vi "EON SubVI.vi"(0 "Image":T1, 5 "Coord details":T2, 7 "Calibrated Image":T1, 11 "error in (no error)":errorcluster, 12 "M ROI":T3) -> (4 "Image Out":T1, 6 "EON outer width":sgl format="%.2f", 8 "EON Presence/Absence":bool, 15 "error out":errorcluster)   [LabVIEW 2019, in "Algorithm.lvclass"]
uses:
  FrameworkOverrides/Algorithm.lvclass
  <vilib>/vision/NI_Vision_Development_Module.lvlib
  <vilib>/vision/Measure.llb/Edge Polarity.ctl
  <vilib>/vision/Measure.llb/Edge Options.ctl
  <vilib>/vision/Image Controls.llb/IMAQ Image.ctl
panel:
  out "Overlay Delay":u64
  out "EON Presence":i32
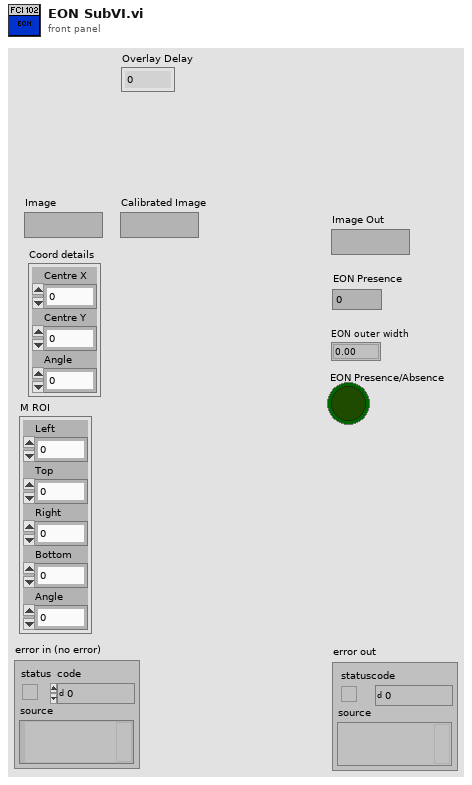
[diagram p1: front panel]
types:
  T1 = typedef "IMAQ Image.ctl" = refnum<image>
  T2 = cluster{"Centre X":dbl, "Centre Y":dbl, "Angle":dbl}
  T3 = cluster{"Left":dbl, "Top":dbl, "Right":dbl, "Bottom":dbl, "Angle":dbl}
  T4 = typedef "Edge Options.ctl" = cluster{"Edge Polarity":T5, "Kernel Size":u32, "Width":u32, "Minimum Edge Strength":sgl, "Interpolation Type":enum32{"Zero Order", "Bilinear", "Quadratic", "Cubic", "Bilinear Fixed"}, "Data Processing Method":enum32{"Average", "Median"}}
  T5 = typedef "Edge Polarity.ctl" = u32
  T6 = typedef "Particle Parameters" = i32
  T7 = cluster{"Measurement Parameter":T6, "Range Lower Value":dbl, "Range Upper Value":dbl, "Range":bool, "Measurement Type":bool}[]
  T8 = typedef "Image Type" = u32
  T9 = typedef "ROI Descriptor" = cluster{"Global Rectangle":i32[], "Contours":cluster{"ID":enum32{"External", "Internal"}, "Type":u32, "Coordinates":i32[]}[]}
  T10 = typedef "Search Line.ctl" = cluster{"Start Point":cluster{"X":sgl, "Y":sgl}, "End Point":cluster{"X":sgl, "Y":sgl}, "Edge Info":T11[], "Edge Map":dbl[], "Calibration Valid":bool}
  T11 = typedef "Edge New.ctl" = cluster{"Location (Pixel)":cluster{"X":sgl, "Y":sgl}, "Location (Real-World)":cluster{"X":sgl, "Y":sgl}, "Distance (Pixel)":dbl, "Distance (Real-World)":dbl, "Strength":dbl, "Noise":dbl, "Rising?":bool}
  T12 = cluster{"Search Lines":T10[], "First Edge Points Array":cluster{"X":sgl, "Y":sgl}[], "Last Edge Points Array":cluster{"X":sgl, "Y":sgl}[]}
  T13 = cluster{"First Edge Point":cluster{"X":sgl, "Y":sgl}, "Search Line First Edge":cluster{"X":sgl, "Y":sgl}}
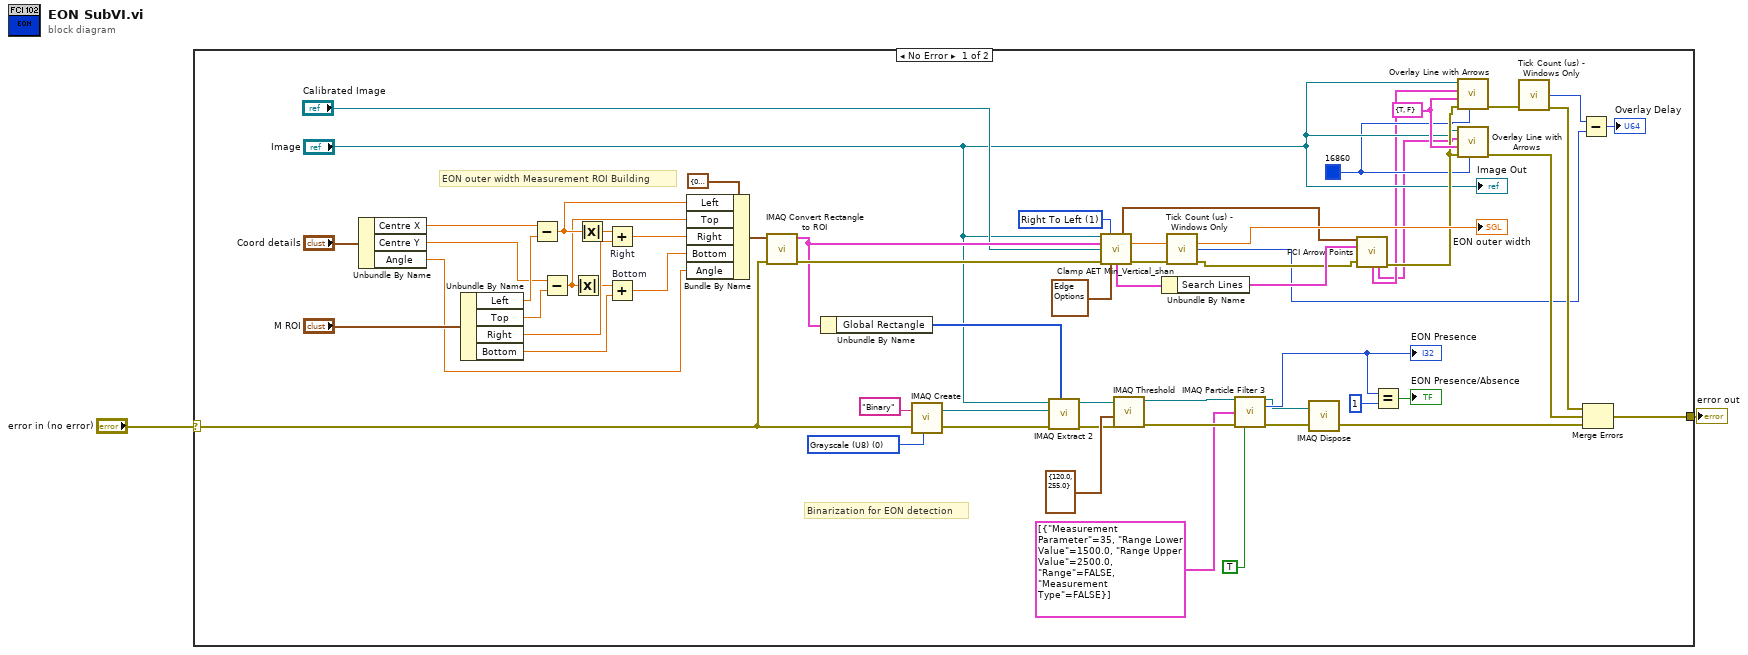
[diagram p0: block diagram]
diagram:
  n1 = case shown="No Error" "error in (no error)" {
    selector: "error in (no error)" -> [w22 w63]
    tunnel: [w21 w63] -> w1
    frame No Error {
      w13 = u32 16860 ("Color")
      w18 = cluster{"Start point":bool, "End point":bool} {"Start point"=TRUE, "End point"=FALSE} ("Arrows")
      w37 = T8 0 items=["Grayscale (U8)", "Grayscale (I16)", "Grayscale (SGL)", "Complex (CSG)", "RGB (U32)", "HSL (U32)", "RGB (U64)", "Grayscale (U16)"] ("Image Type")
      w49 = u16 1 items=["Left To Right", "Right To Left", "Top To Bottom", "Bottom To Top"] ("Scanning axis")
      # "Binarization for EON detection"
      # "EON outer width Measurement ROI Building"
      n2 = Unbundle By Name("Coord details") -> ("Centre X"=w25:dbl, "Centre Y"=w24:dbl, "Angle"=w23:dbl)
      n3 = Unbundle By Name("M ROI") -> ("Left"=w57:dbl, "Top"=w56:dbl, "Right"=w55:dbl, "Bottom"=w54:dbl)
      n4 = Subtract(x=w25, y=w57) -> (x-y=w60:dbl)
      n5 = Subtract(x=w24, y=w56) -> (x-y=w52:dbl)
      n6 = Absolute Value(x=w52) -> (abs(x)=w53:dbl)
      n7 = Absolute Value(x=w60) -> (abs(x)=w62:dbl)
      n8 = Add "Right"(x=w62, y=w55) -> (x+y=w59:dbl)
      n9 = Add "Bottom"(x=w53, y=w54) -> (x+y=w58:dbl)
      n10 = Bundle By Name(cluster=T3 {"Left"=0.0, "Top"=0.0, "Right"=0.0, "Bottom"=0.0, "Angle"=0.0} ("input cluster"), "Left"=w60, "Top"=w52, "Right"=w59, "Bottom"=w58, "Angle"=w23) -> (w51:T3)
      n11 = call "IMAQ Convert Rectangle to ROI"("error in (no error)"=w22, "Rectangle"=w51) -> ("error out"=w50:errorcluster, "ROI Descriptor"=w43:T9)  [unwired: 7 in]
      n12 = Unbundle By Name(w43) -> ("Global Rectangle"=w42:i32[])
      n13 = call "IMAQ Create"("Image Name"="Binary", "Image Type"=w37, "error in (no error)"=w22) -> ("New Image"=w28:T1, "error out"=w33:errorcluster)  [unwired: 2 in]
      n14 = call "IMAQ Extract 2"("Optional Rectangle"=w42, "error in (no error)"=w33, "Image Dst"=w28, "Image Src"="Image") -> ("error out"=w32:errorcluster, "Image Dst Out"=w44:T1)  [unwired: 6 in]
      n15 = call "Clamp AET Min_Vertical_shan.vi"("Image"="Image", "Scanning axis"=w49, "ROI Descriptor"=w43, "Calibrated Image"="Calibrated Image", "error in (no error)"=w50, "Edge Options"=T4 {"Edge Polarity"=0, "Kernel Size"=3, "Width"=3, "Minimum Edge Strength"=50.0, "Interpolation Type"=enum."Zero Order", "Data Processing Method"=enum."Average"}) -> ("Edge Coordinates"=w3:cluster{"X":sgl, "Y":sgl}[], "Distance"=→"EON outer width":sgl, "Overlay Cluster out"=w20:T12, "error out"=w12:errorcluster)  [unwired: 3 in, 3 out]
      n16 = call "IMAQ Threshold"("error in (no error)"=w32, "Range"=cluster{"Lower value":sgl, "Upper value":sgl} {"Lower value"=120.0, "Upper value"=255.0}, "Image Src"=w44) -> ("error out"=w46:errorcluster, "Image Dst Out"=w45:T1)  [unwired: 7 in]
      n17 = Unbundle By Name(w20) -> ("Search Lines"=w19:T10[])
      n18 = call "Tick Count (us) - Windows Only.vi"("error in (no error)"=w12) -> ("micorsecond timer value"=w7:u64, "error out"=w11:errorcluster)  [unwired: 13 in]
      n19 = call "IMAQ Particle Filter 3"("Image Src"=w45, "Selection Values"=T7 [{"Measurement Parameter"=35, "Range Lower Value"=1500.0, "Range Upper Value"=2500.0, "Range"=FALSE, "Measurement Type"=FALSE}], "error in (no error)"=w46, "Reject Border? (F)"=TRUE) -> ("Image Dst Out"=w30:T1, "Number of Particles"=w36:i32, "error out"=w31:errorcluster)  [unwired: 9 in]
      "EON Presence" <- w36
      n20 = call "IMAQ Dispose"("Image"=w30, "error in (no error)"=w31) -> ("error out"=w29:errorcluster)  [unwired: 4 in]
      n21 = call "FCI Arrow Points.vi"("Max Edge Points"=w3, "Search Lines"=w19, "error constant"=w11) -> ("Max first Arrow Line Coord out"=w5:T13, "Max Last Arrow Line Coord out"=w4:T13, "error IO"=w17:errorcluster)  [unwired: 8 in, 2 out]
      n22 = Equal?(x=w36, y=1) -> (x = y?=→"EON Presence/Absence":bool)
      n23 = call <vilib>:"Overlay Line with Arrows.vi"("Color"=w13, "error in (no error)"=w17, "Arrows"=w18, "Line Coordinates"=w5, "Image In"="Image") -> ("error out"=w10:errorcluster)  [unwired: 5 in, 1 out]
      n24 = call <vilib>:"Overlay Line with Arrows.vi"("Color"=w13, "error in (no error)"=w17, "Arrows"=w18, "Line Coordinates"=w4, "Image In"="Image") -> ("error out"=w16:errorcluster)  [unwired: 5 in, 1 out]
      n25 = call "Tick Count (us) - Windows Only.vi"("error in (no error)"=w10) -> ("micorsecond timer value"=w8:u64, "error out"=w9:errorcluster)  [unwired: 13 in]
      n26 = Subtract(x=w8, y=w7) -> (x-y=→"Overlay Delay":u64)
      n27 = Merge Errors(w9, w16, w29) -> (w21:errorcluster)
      "Image Out" <- "Image"
    }
    frame Error {
    }
  }
  "error out" <- w1
